vi "Menu Build Settings Item.vi"() -> (3 "Menu Settings Item":refnum<data-value>)   [LabVIEW 2018, in "LF2R IDE.lvlib" / "LF2R IDE.lvclass"]
uses:
  LF2R IDE.lvclass
  <userlib>/_MGI/Menu Building/MenuItem/MGI_MenuItem.lvclass
  Menu item.ctl
  <userlib>/_MGI/Menu Building/MenuItem/MenuItem.vi
  <userlib>/_MGI/Menu Building/MenuItem/Write Sub-Menus.vi
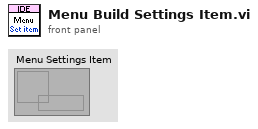
[diagram p1: front panel]
types:
  T1 = typedef "LF2R IDE.lvlib/LF2R IDE.lvclass/Menu Item.ctl" = enum16{"INVALID ITEM", "Open File", "Save File", "Exit", "Preferences"}
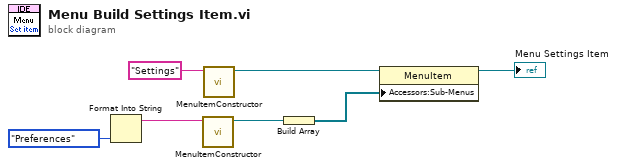
[diagram p0: block diagram]
diagram:
  n1 = Format Into String(Menu_Item."Preferences" ("Menu item")) -> (resulting string=w2:string)  [unwired: 3 in, 1 out]
  n2 = call-poly <userlib>:"MenuItemConstructor.vi"("Text"=w2) -> ("MenuItem"=w5:refnum<data-value>)  [unwired: 9 in, 1 out]
  n3 = call-poly <userlib>:"MenuItemConstructor.vi"("Text"="Settings") -> ("MenuItem"=w7:refnum<data-value>)  [unwired: 9 in, 1 out]
  n4 = Build Array(w5) -> (w4:refnum<data-value>[])
  n5 = property class="MenuItem"(reference=w7, "Accessors:Sub-Menus"=w4) -> (reference out=→"Menu Settings Item":refnum<data-value>)  [unwired: 1 in, 1 out]
